vi "FipsAdjacentLevels.vi"(10 "Levels":i32, 11 "Fips":i32) -> (3 "FipsOut":i32[](array[numeric]))   [LabVIEW 2017]
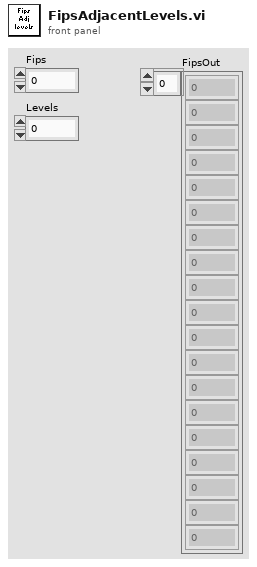
[diagram p1: front panel]
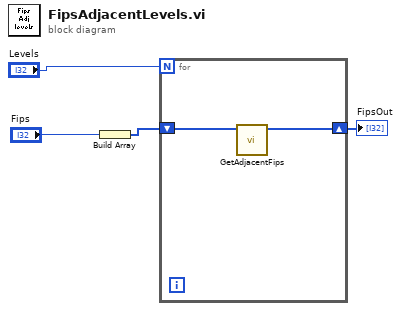
[diagram p0: block diagram]
diagram:
  n1 = Build Array("Fips") -> (w3:i32[])
  n2 = for {
    N: "Levels" -> [_]
    shift-right: [w5] -> w1
    shift-left: w3 -> [w6]
    n3 = call "GetAdjacentFips.vi"("FipsIn"=w6) -> ("FipsOut"=w5:i32[])  [unwired: 10 in]
  }
  "FipsOut" <- w1
